vi "init_plot.vi"(2 "1-D Array of Real 4":dbl[](array[numeric])=[10.0, 20.0], 3 "1-D Array of Real 3":dbl[](array[numeric])=[10.0, 30.0, 150.0, 180.0], 4 "1-D Array of Real 2":dbl[](array[numeric])=[10.0, 20.0], 5 "1-D Array of Real":dbl[](array[numeric])=[10.0, 30.0, 150.0, 180.0]) -> ()   [LabVIEW 2012]
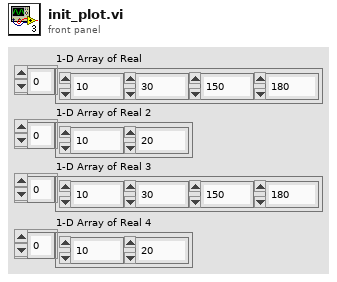
[diagram p1: front panel]
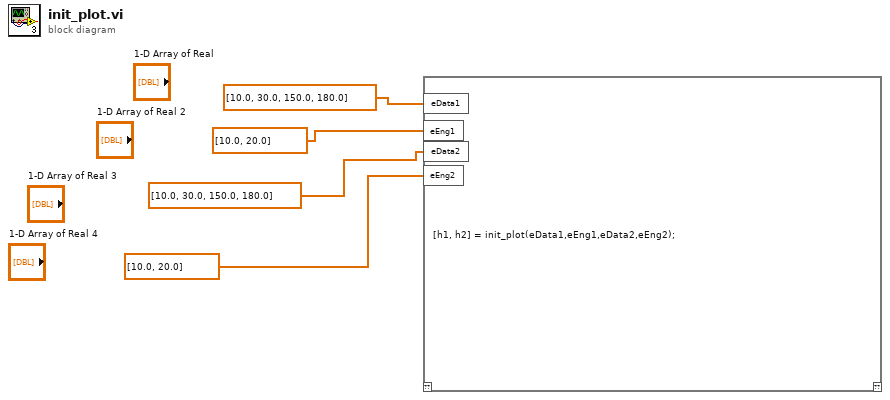
[diagram p0: block diagram]
diagram:
  n1 = script code="[h1, h2] = init_plot(eData1,eEng1,eData2,eEng2);"("eData1"=dbl[] [10.0, 30.0, 150.0, 180.0] ("1-D Array of Real"), "eEng1"=dbl[] [10.0, 20.0] ("1-D Array of Real"), "eData2"=dbl[] [10.0, 30.0, 150.0, 180.0] ("1-D Array of Real"), "eEng2"=dbl[] [10.0, 20.0] ("1-D Array of Real")) -> ()  [unwired: 1 in, 1 out]
